vi "Initilaize Views.vi"(8 "error in (no error)":errorcluster, 11 "Example Controller in":refnum<class "Example Controller.lvclass">) -> (0 "error out":errorcluster, 3 "Example Controller out":refnum<class "Example Controller.lvclass">)   [LabVIEW 2023, in "Example GUI View.lvlib" / "Example Controller.lvclass"]
uses:
  Example Controller.lvclass
  Example GUI Container/Example GUI Container.lvclass
  View/View.lvclass/View.ctl
  Example Controller.lvclass/Example Controller.ctl
  View/properties/Write Name.vi
  Example Controller/Example Controller/Example Controller.lvclass
  Controller/Controller.lvclass
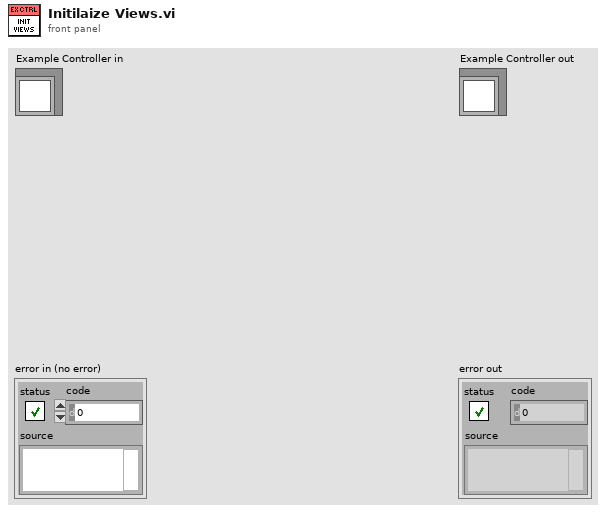
[diagram p1: front panel]
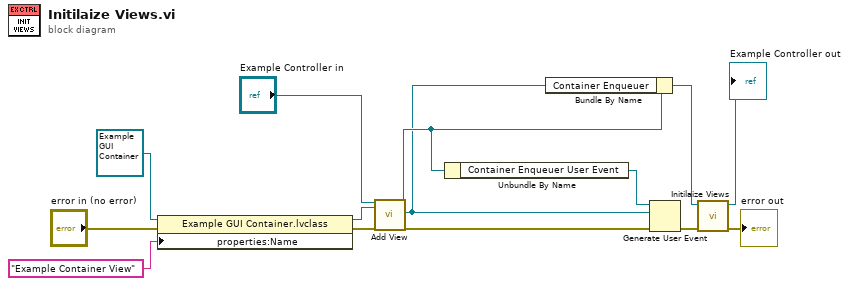
[diagram p0: block diagram]
diagram:
  n1 = property class="Example GUI Container.lvclass"(reference=refnum<class "Example GUI Container.lvclass"> refnum ("Example GUI View Actor.lvlib:Example GUI Container.lvclass"), error in="error in (no error)", "properties:Name"="Example Container View" ("Debug Alias")) -> (reference out=w12:refnum<class "Example GUI Container.lvclass">, error out=w10:errorcluster)
  n2 = call "Add View.vi"("Controller in"="Example Controller in", "View Actor"=w12, "error in (no error)"=w10) -> ("Controller out"=w3:refnum<class "Example Controller.lvclass">, "View Enqueuer"=w1:refnum<class "Message Enqueuer.lvclass">, "error out"=w6:errorcluster)  [unwired: 14 in]
  n3 = Unbundle By Name(w3) -> ("Container Enqueuer User Event"=w2:refnum<user-event>)
  n4 = Bundle By Name(cluster=w3, "Container Enqueuer"=w1) -> (w5:refnum<class "Example Controller.lvclass">)
  n5 = Generate User Event(user event=w2, event data cluster=w1, error in=w6) -> (error out=w4:errorcluster)  [unwired: 1 in, 1 out]
  n6 = call-parent "Initilaize Views.vi"("error in (no error)"=w4, "Example Controller in"=w5) -> ("error out"=→"error out":errorcluster, "Example Controller out"=→"Example Controller out":refnum<class "Example Controller.lvclass">)  [unwired: 8 in]
